vi "Parse Data Filename.vi"(11 "Filename":string) -> (0 "Suffix":string, 1 "Run":i32, 2 "Site":i32, 3 "Exp":string, 4 "extension":string)   [LabVIEW 2020]
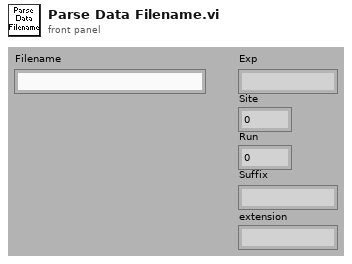
[diagram p1: front panel]
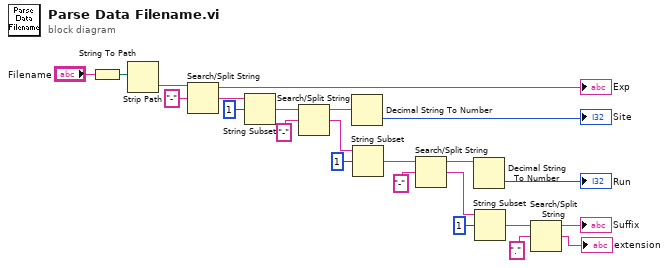
[diagram p0: block diagram]
diagram:
  n1 = String To Path(string="Filename") -> (path=w2:path)
  n2 = Strip Path(path=w2) -> (name=w1:string)  [unwired: 1 out]
  n3 = Search/Split String(string=w1, search string/char (-)="-") -> (substring before match=→"Exp":string, match + rest of string=w13:string)  [unwired: 1 in, 1 out]
  n4 = String Subset(string=w13, offset (0)=1) -> (substring=w11:string)  [unwired: 1 in]
  n5 = Search/Split String(string=w11, search string/char (-)="-") -> (substring before match=w21:string, match + rest of string=w9:string)  [unwired: 1 in, 1 out]
  n6 = Decimal String To Number(string=w21) -> (number=→"Site":i32)  [unwired: 2 in, 1 out]
  n7 = String Subset(string=w9, offset (0)=1) -> (substring=w8:string)  [unwired: 1 in]
  n8 = Search/Split String(string=w8, search string/char (-)="-") -> (substring before match=w18:string, match + rest of string=w6:string)  [unwired: 1 in, 1 out]
  n9 = Decimal String To Number(string=w18) -> (number=→"Run":i32)  [unwired: 2 in, 1 out]
  n10 = String Subset(string=w6, offset (0)=1) -> (substring=w5:string)  [unwired: 1 in]
  n11 = Search/Split String(string=w5, search string/char (-)=".") -> (substring before match=→"Suffix":string, match + rest of string=→"extension":string)  [unwired: 1 in, 1 out]
